vi "VideoCapture Read.vi"(8 "error in (no error)":errorcluster, 10 "Image":T1, 11 "VideoCapture in":refnum<class "VideoCapture.lvclass">) -> (0 "error out":errorcluster, 1 "Success":bool, 2 "Image out":T1, 3 "VideoCapture out":refnum<class "VideoCapture.lvclass">)   [LabVIEW 2020, in "OpenLvVision_OpenCv.lvlib" / "VideoCapture.lvclass"]
doc: "Grabs, decodes and returns the next video frame."
uses:
  VideoCapture.lvclass
  C:/Users/lukas/Downloads/OpenLvVision_OpenCv/SourceCode/LabView/OpenLvVision_OpenCv/_LvHelpers/EdvrObject/EdvrObject.lvclass
  <vilib>/vision/Image Controls.llb/IMAQ Image.ctl
  _LvHelpers/EdvrObject/EdvrObject.lvclass/EdvrObject.ctl
  OpenLvVision_OpenCv.lvlib
  _LvHelpers/EdvrObject/EdvrObject.lvclass
  Dlls/OlvOpenCvWrapper.dll
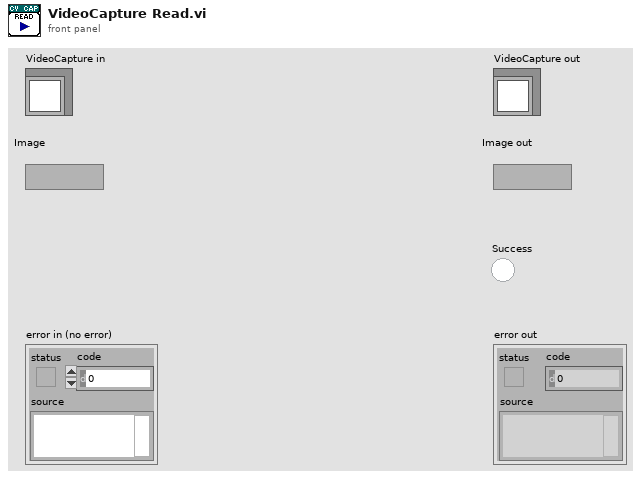
[diagram p1: front panel]
types:
  T1 = typedef "IMAQ Image.ctl" = refnum<image>
  T2 = typedef "OpenLvVision_OpenCv.lvlib/EdvrObject.lvclass/Edvr.ctl" = refnum<data-value>
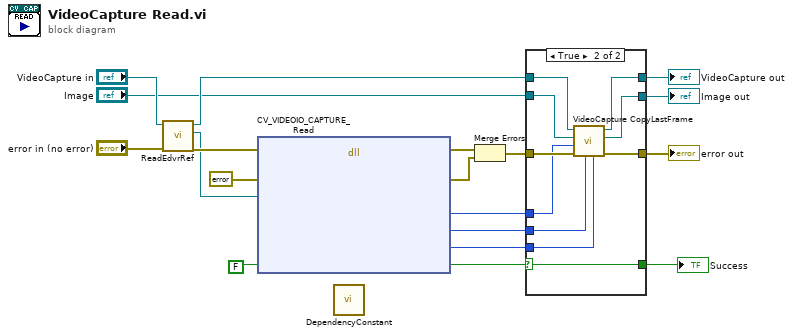
[diagram p0: block diagram]
diagram:
  n1 = call "ReadEdvrRef.vi"("error in (no error)"="error in (no error)", "EdvrObject in"="VideoCapture in") -> ("error out"=w18:errorcluster, "Edvr"=w17:T2, "EdvrObject out"=w10:refnum<class "VideoCapture.lvclass">)  [unwired: 7 in]
  n2 = dll-call lib="C:/Users/lukas/Downloads/OpenLvVision_OpenCv/SourceCode/LabView/OpenLvVision_OpenCv/Dlls/OlvOpenCvWrapper.dll" fn="CV_VIDEOIO_CAPTURE_Read"(error in=w18, "Error"=errorcluster {"status"=FALSE, "code"=0, "source"=""} ("error out"), "edvrRef"=w17, "result"=FALSE) -> (error out=w16:errorcluster, "Error"=w15:errorcluster, "width"=w3:i32, "height"=w2:i32, "imageType"=w1:i32, "result"=w11:bool)  [unwired: 7 in, 1 out]
  n3 = call "DependencyConstant.vi"() -> ()  [unwired: 12 in]
  n4 = Merge Errors(w16, w15) -> (w13:errorcluster)
  n5 = case shown="True" w11 {
    selector: w11 -> [w20 w29]
    tunnel: w13 -> [w21 w28]
    tunnel: [w21 w33] -> w12
    tunnel: w10 -> [w23 w32]
    tunnel: [w23 w31] -> w9
    tunnel: [w22 w30] -> w8
    tunnel: "Image" -> [w22 w27]
    tunnel: [w20 w29] -> w5
    tunnel: w3 -> [_ w26]
    tunnel: w2 -> [_ w25]
    tunnel: w1 -> [_ w24]
    frame False {
    }
    frame True {
      n6 = call "VideoCapture CopyLastFrame.vi"("Image Type"=w24, "height"=w25, "error in (no error)"=w28, "width"=w26, "Image"=w27, "VideoCapture in"=w32) -> ("error out"=w33:errorcluster, "Image"=w30:T1, "VideoCapture out"=w31:refnum<class "VideoCapture.lvclass">)  [unwired: 3 in]
    }
  }
  "error out" <- w12
  "VideoCapture out" <- w9
  "Image out" <- w8
  "Success" <- w5
